vi "QTrkMinimalTest.vi"() -> ()   [LabVIEW 2015]
uses:
  QTrkLVBinding/QTrkSettings.ctl
  QTrkLVBinding/QTrkDLL.vi
panel:
  in  "QTrk Settings":T1={"Image width"=150, "Image height"=150, "Number of threads (CPU based)"=-1, "CUDA Device"=128, "COM Background correction factor"=2.0, "ZLUT MinRadius"=5.0, "ZLUT Radial sample density"=40.0, "ZLUT Angular sample density"=128.0, "ZLUT ROI Coverage"=32.0, "QI Iterations"=4, "QI MinRadius"=5.0, "QI Radial sample density"=32.0, "QI Angular sample density"=40.0, "QI ROI Coverage"=-1.0, "QI Angular Step \nIteration Factor"=32.0, "XCOR Profile Length"=32, "XCOR Profile Width"=2, "XCOR Iterations"=5, "Gaussian 2D Fit Iterations"=8, "Gaussian 2D Sigma (pixels)"=3.0, "Downsample"=0}
  # "-2: Use all devices\n-1: Use best device"
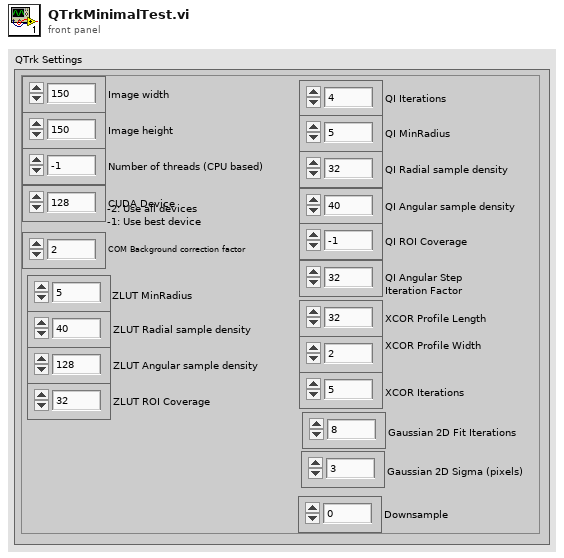
[diagram p1: front panel]
types:
  T1 = typedef "QTrkSettings.ctl" = cluster{"Image width":i32, "Image height":i32, "Number of threads (CPU based)":i32, "CUDA Device":i32, "COM Background correction factor":sgl, "ZLUT MinRadius":sgl, "ZLUT Radial sample density":sgl, "ZLUT Angular sample density":sgl, "ZLUT ROI Coverage":sgl, "QI Iterations":i32, "QI MinRadius":sgl, "QI Radial sample density":sgl, "QI Angular sample density":sgl, "QI ROI Coverage":sgl, "QI Angular Step \nIteration Factor":sgl, "XCOR Profile Length":i32, "XCOR Profile Width":i32, "XCOR Iterations":i32, "Gaussian 2D Fit Iterations":i32, "Gaussian 2D Sigma (pixels)":sgl, "Downsample":i32}
  T2 = typedef "QTrkInstance.ctl" = cluster{"QTrk Pointer":u64}
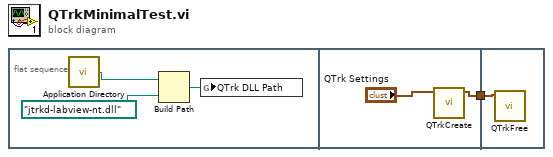
[diagram p0: block diagram]
diagram:
  n1 = flat-sequence {
    tunnel: [w5] -> w1
    tunnel: w1 -> [w7]
    frame #0 {
      n2 = call <vilib>:"Application Directory.vi"() -> ("Application Directory"=w2:path)
      n3 = Build Path(base path=w2, name or relative path=path "jtrkd-labview-nt.dll") -> (appended path=w3:path)
      n4 = global write "QTrkDLL.vi" "QTrk DLL Path"(w3) -> ()
    }
    frame #1 {
      n5 = call "QTrkCreate.vi"("QTrk Settings"="QTrk Settings") -> ("QTrk Instance"=w5:T2)  [unwired: 4 in, 2 out]
    }
    frame #2 {
      n6 = call "QTrkFree.vi"("QTrk Instance"=w7) -> ()  [unwired: 6 in, 1 out]
    }
  }
